vi "oa_CIC Interpolation Filter.vi"(7 "reset? (True)":bool=TRUE, 8 "error in (no error)":errorcluster, 9 "CIC filter settings":T1(array[cluster]), 11 "X":dbl[](array[numeric]) format="%.2f") -> (0 "error out":errorcluster, 3 "Y":dbl[](array[numeric]) format="%.2f")   [LabVIEW 2017, in "SoundVib_Resampling.lvlib"]
uses:
  <vilib>/addons/Sound and Vibration/Order Analysis/Resample Order Tracking/SoundVib_Resampling.lvlib
  <vilib>/addons/Sound and Vibration/Order Analysis/Resample Order Tracking/SubVIs/oa_CIC Filter Length.vi
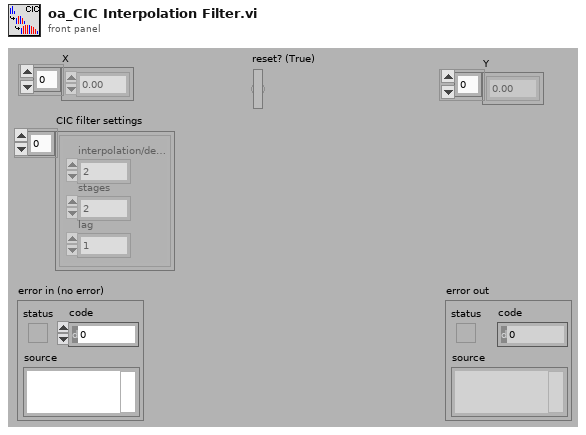
[diagram p1: front panel]
types:
  T1 = cluster{"interpolation/decimation factor":i32, "stages":i32, "lag":i32}[]
  T2 = cluster{"corrected lengths":i32[], "initH":cluster{"t":dbl[]}[]}
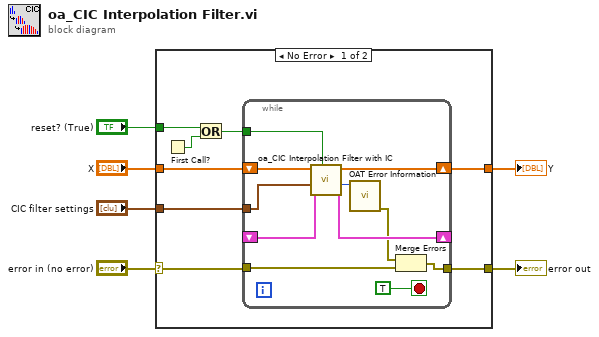
[diagram p0: block diagram]
diagram:
  n1 = case shown="No Error" "error in (no error)" {
    selector: "error in (no error)" -> [w10 w26]
    tunnel: "CIC filter settings" -> [w14 _]
    tunnel: "X" -> [w13 _]
    tunnel: [w12 _] -> w4
    tunnel: [w11 w26] -> w2
    tunnel: "reset? (True)" -> [w8 _]
    frame No Error {
      n2 = First Call?() -> (First Call?: T/F=w9:bool)
      n3 = Or(x=w8, y=w9) -> (x .or. y?=w7:bool)
      n4 = while {
        tunnel: w14 -> [w20]
        tunnel: [w24] -> w11
        tunnel: w7 -> [w18]
        tunnel: w10 -> [w23]
        shift-right: [w22] -> _
        shift-left: _ -> [w21]
        shift-right: [w17] -> w12
        shift-left: w13 -> [w19]
        stop <- TRUE stop-if-true
        n5 = call <vilib>:"oa_CIC Interpolation Filter with IC.vi"("reset? (True)"=w18, "initial conditions"=w21, "CIC filter settings"=w20, "X"=w19) -> ("final conditions"=w22:T2, "error"=w16:i32, "Y"=w17:dbl[])  [unwired: 5 in]
        n6 = call <vilib>:"OAT Error Information.vi"("error code"=w16) -> ("error out"=w15:errorcluster)  [unwired: 6 in]
        n7 = Merge Errors(w15, w23) -> (w24:errorcluster)
      }
    }
    frame Error {
    }
  }
  "Y" <- w4
  "error out" <- w2
